vi "image_data_to_I32.vi"(1 "Data In":cluster{"X":dbl, "Y":dbl}[][](array[cluster])) -> (0 "Data Out":cluster{"X":i32, "Y":i32}[][](array[cluster]))   [LabVIEW 2017]
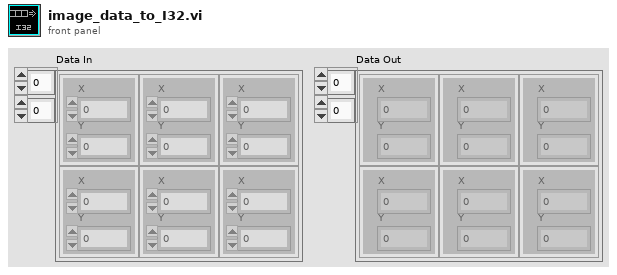
[diagram p1: front panel]
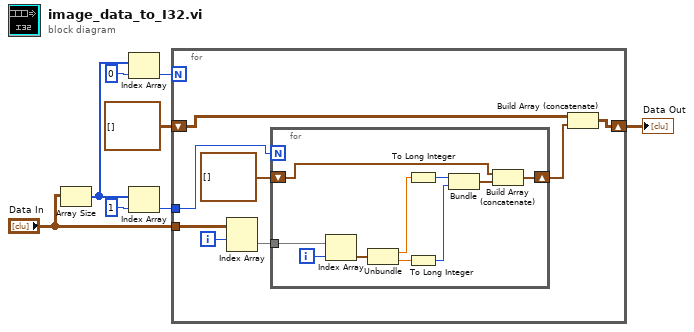
[diagram p0: block diagram]
diagram:
  n1 = Array Size(array="Data In") -> (size(s)=w4:i32[])
  n2 = Index Array(array=w4, index=0) -> (element=w7:i32)
  n3 = Index Array(array=w4, index=1) -> (element=w3:i32)
  n4 = for {
    N: w7 -> [_]
    tunnel: "Data In" -> [w16]
    tunnel: w3 -> [w14]
    shift-right: [w10] -> w2
    shift-left: cluster{i32, i32}[][] [] -> [w12]
    i -> [w15]
    n5 = Index Array(array=w16, index (row)=w15) -> (element=w13:cluster{"X":dbl, "Y":dbl}[])  [unwired: 1 in]
    n6 = for {
      N: w14 -> [_]
      shift-right: [w25] -> w11
      shift-left: cluster{i32, i32}[] [] -> [w26]
      tunnel: w13 -> [w24]
      i -> [w23]
      n7 = Index Array(array=w24, index=w23) -> (element=w22:cluster{"X":dbl, "Y":dbl})
      n8 = Unbundle(w22) -> ("X"=w21:dbl, "Y"=w18:dbl)
      n9 = To Long Integer(number=w21) -> (32bit integer=w19:i32)
      n10 = To Long Integer(number=w18) -> (32bit integer=w20:i32)
      n11 = Bundle(w19, w20) -> (w17:cluster{i32, i32})  [unwired: 1 in]
      n12 = Build Array (concatenate)(w26, w17) -> (w25:cluster{i32, i32}[])
    }
    n13 = Build Array (concatenate)(w12, w11) -> (w10:cluster{i32, i32}[][])
  }
  "Data Out" <- w2
